vi "Import ESI File.vi"(8 "error in":errorcluster) -> (0 "error out":errorcluster)   [LabVIEW 2019, in "SEECD System Explorer.lvlib"]
uses:
  SEECD System Explorer.lvlib
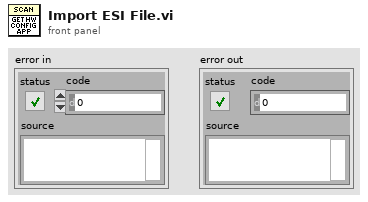
[diagram p1: front panel]
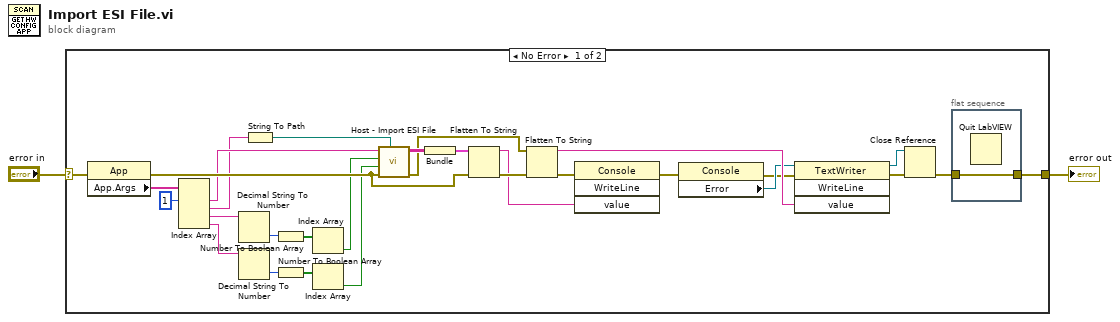
[diagram p0: block diagram]
diagram:
  n1 = case shown="No Error" "error in" {
    selector: "error in" -> [w30 w33]
    tunnel: [w28 w33] -> w2
    frame No Error {
      n2 = property class="App"(error in=w30) -> (error out=w14:errorcluster, "App.Args"=w31:string[])  [unwired: 1 in, 1 out]
      n3 = Index Array(array=w31, index #1=1 ("index")) -> (element #1=w13:string, element #2=w12:string, element #3=w10:string, element #4=w16:string)  [unwired: 3 in]
      n4 = Decimal String To Number(string=w10) -> (number=w9:i32)  [unwired: 2 in, 1 out]
      n5 = Decimal String To Number(string=w16) -> (number=w8:i32)  [unwired: 2 in, 1 out]
      n6 = String To Path(string=w12) -> (path=w11:path)
      n7 = Number To Boolean Array(number=w9) -> (Boolean array=w7:bool[])
      n8 = Number To Boolean Array(number=w8) -> (Boolean array=w5:bool[])
      n9 = Index Array(array=w7) -> (element=w6:bool)  [unwired: 1 in]
      n10 = Index Array(array=w5) -> (element=w4:bool)  [unwired: 1 in]
      n11 = call "Host - Import ESI File.vi"("Select a device profile or file path"=w11, "error in"=w14, "Import to RT target"=w4, "Import to host PC"=w6, "Target IP Address"=w13) -> ("error out"=w3:errorcluster, "result out"=w15:string[][])  [unwired: 5 in]
      n12 = Bundle("result out"=w15) -> (w17:cluster{"result out":string[][]})  [unwired: 1 in]
      n13 = Flatten To String(anything=w17, error in (no error)=w14) -> (data string=w25:string, error out=w27:errorcluster)  [unwired: 2 in, 1 out]
      n14 = Flatten To String(anything=w3, error in (no error)=w27) -> (data string=w24:string, error out=w26:errorcluster)  [unwired: 2 in, 1 out]
      n15 = invoke class="Console" method="WriteLine"(error in=w26, "value"=w25) -> (error out=w18:errorcluster)  [unwired: 2 in, 3 out]
      n16 = property class="Console"(error in=w18) -> (error out=w19:errorcluster, "Error"=w23:refnum<k24>)  [unwired: 1 in, 1 out]
      n17 = invoke class="TextWriter" method="WriteLine"(reference=w23, error in=w19, "value"=w24) -> (reference out=w21:refnum<k24>, error out=w22:errorcluster)  [unwired: 1 in, 2 out]
      n18 = Close Reference(reference=w21, error in (no error)=w22) -> (error out=w20:errorcluster)
      n19 = flat-sequence {
        tunnel: w20 -> [w32]
        tunnel: [w32] -> w28
        frame #0 {
          n20 = Quit LabVIEW() -> ()  [unwired: 1 in]
        }
      }
    }
    frame Error {
    }
  }
  "error out" <- w2
